vi "run.vi"(8 "error in (no error)":errorcluster, 11 "dotnet_system_exec in":refnum<class "dotnet_system_exec.lvclass">) -> (0 "error out":errorcluster, 3 "dotnet_system_exec out":refnum<class "dotnet_system_exec.lvclass">)   [LabVIEW 2020, in "JKI dotNET System Exec.lvlib" / "dotnet_system_exec.lvclass"]
doc: "Runs the .NET System Process as configured with the @create method\n\n-----------------------------------------------\nJKI .NET System Exec 1.0.0.6\nJavier Ruiz - JKI\nCopyright (c) 2021, JKI\njki.net"
uses:
  dotnet_system_exec.lvclass
  dotnet_system_exec.lvclass/dotnet_system_exec.ctl
  output_callback.vi
  process_exit_callback.vi
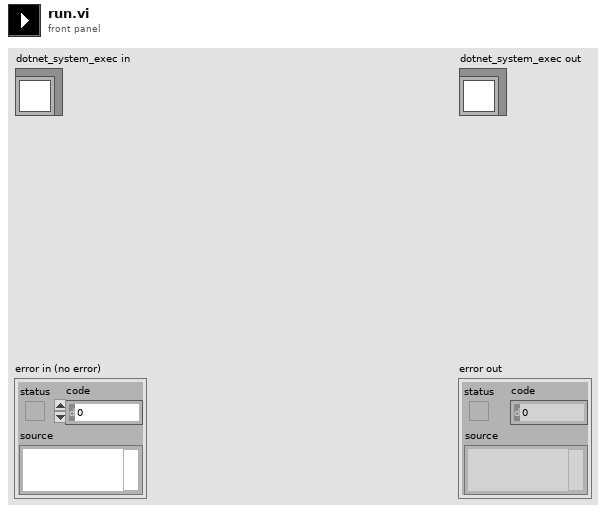
[diagram p1: front panel]
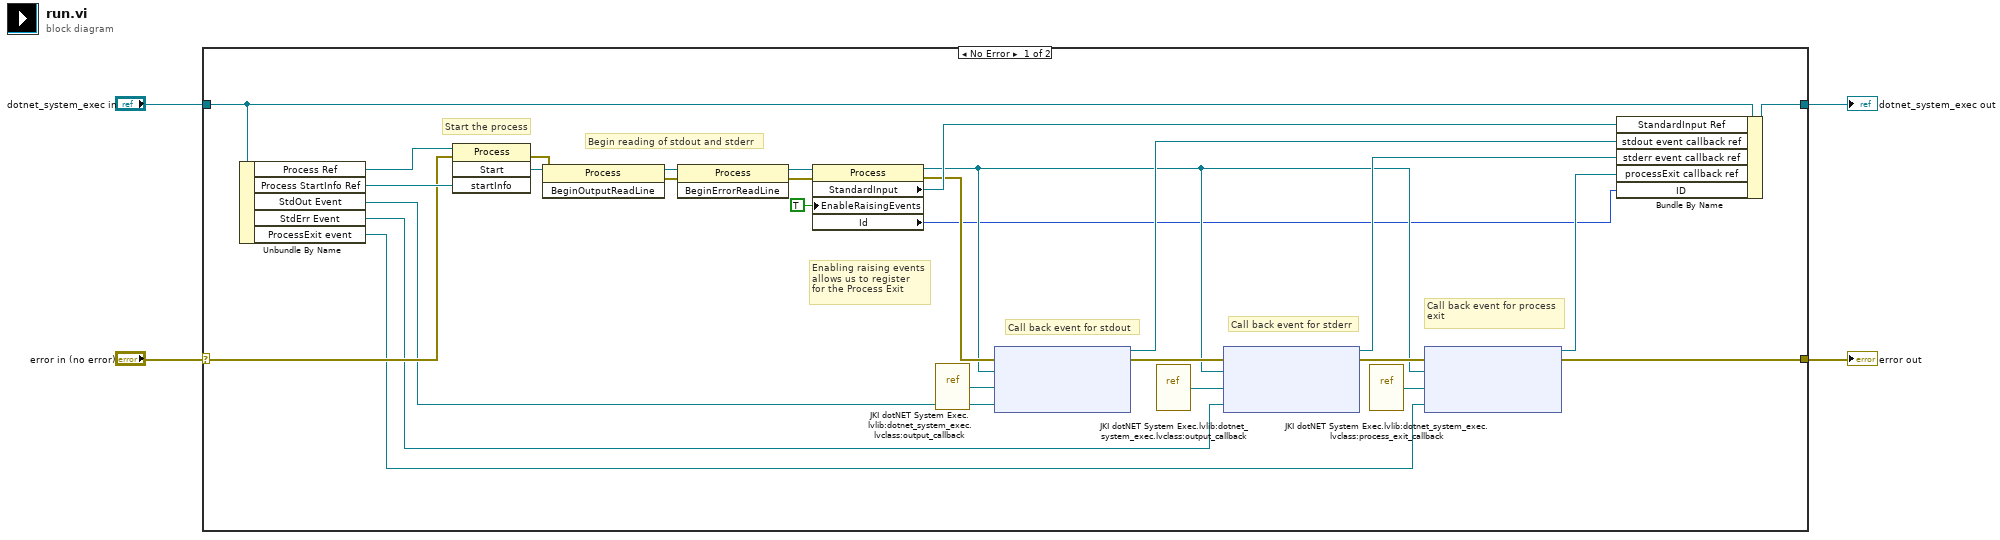
[diagram p0: block diagram]
diagram:
  n1 = case shown="No Error" "error in (no error)" {
    selector: "error in (no error)" -> [w24 w34]
    tunnel: [w9 w34] -> w3
    tunnel: [w17 w33] -> w1
    tunnel: "dotnet_system_exec in" -> [w23 w33]
    frame No Error {
      # "Call back event for process\nexit"
      # "Enabling raising events\nallows us to register\nfor the Process Exit"
      # "Call back event for stderr"
      # "Call back event for stdout"
      # "Begin reading of stdout and stderr"
      # "Start the process"
      n2 = Unbundle By Name(w23) -> ("Process Ref"=w30:refnum<k24>, "Process StartInfo Ref"=w29:refnum<k24>, "StdOut Event"=w21:refnum<user-event>, "StdErr Event"=w20:refnum<user-event>, "ProcessExit event"=w8:refnum<user-event>)
      n3 = invoke class="Process" method="Start"(reference=w30, error in=w24, "startInfo"=w29) -> (error out=w28:errorcluster, "Start"=w27:refnum<k24>)  [unwired: 1 in, 2 out]
      n4 = invoke class="Process" method="BeginOutputReadLine"(reference=w27, error in=w28) -> (reference out=w32:refnum<k24>, error out=w31:errorcluster)  [unwired: 1 in, 1 out]
      n5 = invoke class="Process" method="BeginErrorReadLine"(reference=w32, error in=w31) -> (reference out=w26:refnum<k24>, error out=w25:errorcluster)  [unwired: 1 in, 1 out]
      n6 = property class="Process"(reference=w26, error in=w25, "EnableRaisingEvents"=TRUE) -> (reference out=w10:refnum<k24>, error out=w19:errorcluster, "StandardInput"=w22:refnum<k24>, "Id"=w5:i32)
      n7 = vi-ref "JKI dotNET System Exec.lvlib:dotnet_system_exec.lvclass:output_callback.vi"() -> ("vi reference"=w16:refnum<vi>)
      n8 = node(w19, w10, w16, w21) -> (w13:refnum<k27>, w18:errorcluster)  [unwired: 1 in]
      n9 = vi-ref "JKI dotNET System Exec.lvlib:dotnet_system_exec.lvclass:output_callback.vi"() -> ("vi reference"=w15:refnum<vi>)
      n10 = node(w18, w10, w15, w20) -> (w12:refnum<k27>, w11:errorcluster)  [unwired: 1 in]
      n11 = vi-ref "JKI dotNET System Exec.lvlib:dotnet_system_exec.lvclass:process_exit_callback.vi"() -> ("vi reference"=w7:refnum<vi>)
      n12 = node(w11, w10, w7, w8) -> (w6:refnum<k27>, w9:errorcluster)  [unwired: 1 in]
      n13 = Bundle By Name(cluster=w23, "StandardInput Ref"=w22, "stdout event callback ref"=w13, "stderr event callback ref"=w12, "processExit callback ref"=w6, "ID"=w5) -> (w17:refnum<class "dotnet_system_exec.lvclass">)
    }
    frame Error {
    }
  }
  "error out" <- w3
  "dotnet_system_exec out" <- w1
